vi "Create Action Point.vi"(8 "error in":errorcluster, 9 "Action Point Config from JSON":refnum<class "Config from JSON.lvclass">, 10 "IVritual Instrument":refnum<class "IVirtual Instrument.lvclass">, 11 "Alarming Strategy in":refnum<class "Alarming Actor Strategy.lvclass">) -> (0 "error out":errorcluster, 2 "Action Point out":refnum<class "Action Point.lvclass">, 3 "Alarming Strategy out":refnum<class "Alarming Actor Strategy.lvclass">)   [LabVIEW 2024, in "Alarming Actor Strategy.lvclass"]
uses:
  Alarming Actor Strategy.lvclass
  Alarming Actor Strategy.lvclass/Alarming Actor Strategy.ctl
  Action Point/Action Point.lvclass/Action Point.ctl
  Alarming-Actor/Source/Alarming Actor/Alarming Actor Messages/Add Entry Msg/Add Entry Msg.lvclass/Add Entry Msg.ctl
  <vilib>/ActorFramework/Message Enqueuer/Message Enqueuer.lvclass/Message Enqueuer.ctl
  Action Point/Action Point.lvclass
  Alarming-Actor/Source/Alarming Actor/Alarming Actor Messages/Add Entry Msg/Add Entry Msg.lvclass
  Config from JSON/Config from JSON.lvclass
  D:/git/HAL/Source/Config from JSON/Config from JSON.lvclass
  D:/git/HAL/Source/Interfaces/IConfiguration/IConfiguration.lvclass
  Interfaces/IVirtual Instrument/IVirtual Instrument.lvclass
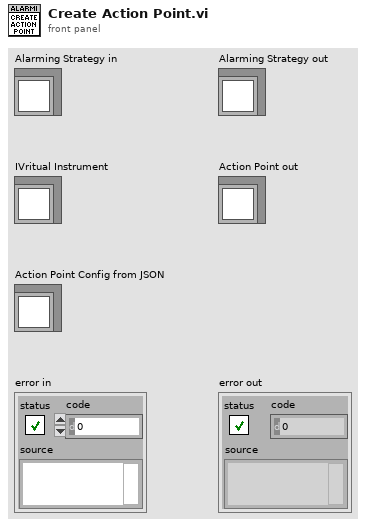
[diagram p1: front panel]
types:
  T1 = cluster{"Hi-Hi":dbl, "Hi":dbl, "Lo":dbl, "Lo-Lo":dbl}
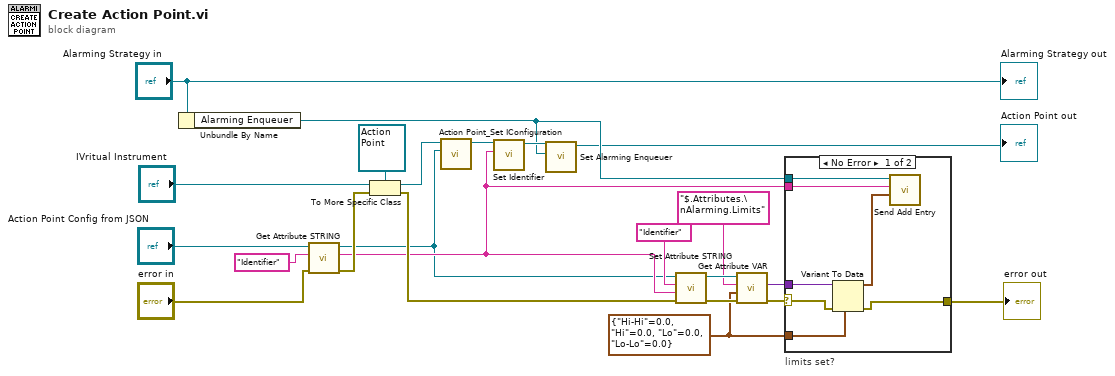
[diagram p0: block diagram]
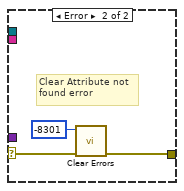
[diagram p2: hidden frame]
diagram:
  w10 = T1 {"Hi-Hi"=0.0, "Hi"=0.0, "Lo"=0.0, "Lo-Lo"=0.0}
  n1 = Unbundle By Name("Alarming Strategy in") -> ("Alarming Enqueuer"=w5:refnum<class "Message Enqueuer.lvclass">)
  n2 = call-dynamic "Get Attribute STRING.vi"("error in"="error in", "Attribute"="Identifier", "ConfigFromJSON in"="Action Point Config from JSON") -> ("error out"=w19:errorcluster, "Value"=w4:string, "ConfigFromJSON out"=w2:refnum<class "Config from JSON.lvclass">)  [unwired: 6 in]
  n3 = To More Specific Class(target class=refnum<class "Action Point.lvclass"> refnum ("Action Point.lvclass"), reference="IVritual Instrument", error in=w19) -> (specific class reference=w21:refnum<class "Action Point.lvclass">, error out=w6:errorcluster)
  n4 = call "Action Point_Set IConfiguration.vi"("IConfiguration"=w2, "Action Point in"=w21) -> ("Action Point out"=w20:refnum<class "Action Point.lvclass">)  [unwired: 9 in]
  n5 = call "Set Identifier.vi"("Identifier"=w4, "Action Point in"=w20) -> ("Action Point out"=w17:refnum<class "Action Point.lvclass">)  [unwired: 9 in]
  n6 = call "Set Alarming Enqueuer.vi"("Alarming Enqueuer"=w5, "Action Point in"=w17) -> ("Action Point out"=→"Action Point out":refnum<class "Action Point.lvclass">)  [unwired: 9 in]
  n7 = call-dynamic "Set Attribute STRING.vi"("error in"=w6, "Value"=w4, "Path"="Identifier", "Config from JSON in"=w2) -> ("error out"=w14:errorcluster, "Config from JSON out"=w12:refnum<class "Config from JSON.lvclass">)  [unwired: 6 in]
  n8 = call-dynamic "Get Attribute VAR.vi"("error in"=w14, "Data Type and Default Value"=w10, "Attribute"="$.Attributes.\nAlarming.Limits", "ConfigFromJSON in"=w12) -> ("error out"=w8:errorcluster, "Value"=w9:variant)  [unwired: 5 in, 1 out]
  n9 = case "limits set?" shown="No Error" w8 {
    selector: w8 -> [w25 w33]
    tunnel: w5 -> [w30 _]
    tunnel: w4 -> [w29 _]
    tunnel: w10 -> [w28 _]
    tunnel: w9 -> [w27 _]
    tunnel: [w24 w32] -> w3
    frame No Error {
      n10 = Variant To Data(error in=w25, type=w28, Variant=w27) -> (data=w26:T1, error out=w24:errorcluster)
      n11 = call "Send Add Entry.vi"("Limits"=w26, "Identifier"=w29, "Message Enqueuer"=w30) -> ()  [unwired: 7 in, 2 out]
    }
    frame Error {
      # "Clear Attribute not\nfound error"
      n12 = call <vilib>:"Clear Errors.vi"("error in (no error)"=w33, "specific error code to clear (0: all)"=-8301) -> ("error out"=w32:errorcluster)  [unwired: 4 in, 1 out]
    }
  }
  "error out" <- w3
  "Alarming Strategy out" <- "Alarming Strategy in"
